vi "Robot Global Data.vi"() -> ()   [LabVIEW 2016]
doc: "This global VI can contain as many global variables as you need. Place a control on the panel, give it a good name. To read or write to it from a VI, drag the icon to the diagram of that VI. You can also drag from the project. Click on the node to change which global you access. You shouldn't have multiple locations writing to a global or it will cause a race-condition."
uses:
  <vilib>/Rock Robotics/WPI/Camera/WPI_CameraImageSize.ctl
  <vilib>/Rock Robotics/WPI/DriverStation/WPI_DriverStationRobotMode2.ctl
panel:
  in  "Robot Enabled":bool
  in  "AutoConstants":T1
  in  "ClimberSpeed":dbl
  in  "IntakeSpeed":dbl
  in  "RightEncoder":dbl
  in  "LeftEncoder":dbl
  in  "Poses":T2(array[cluster])
  in  "Location":cluster{"x":dbl, "y":dbl}
  in  "Angle":dbl
  in  "Diagnostic Message":string
  out "Gear Data":T3
  out "Peg Data":T3
  in  "Vision Target":enum16{"Pegs", "Gears"}(ring)
  in  "RightValue":dbl
  in  "LeftValue":dbl
  in  "ArmState":enum16{"Up", "Down"}(ring)
  in  "PincherState":enum16{"Open", "Close"}(ring)
  in  "Refnums":string[](array[string])
  in  "Robot Mode":T4
  in  "image size":T5=enum."320x240"
  in  "Enable Vision":bool
  # "Drive Base"
  # "Vision"
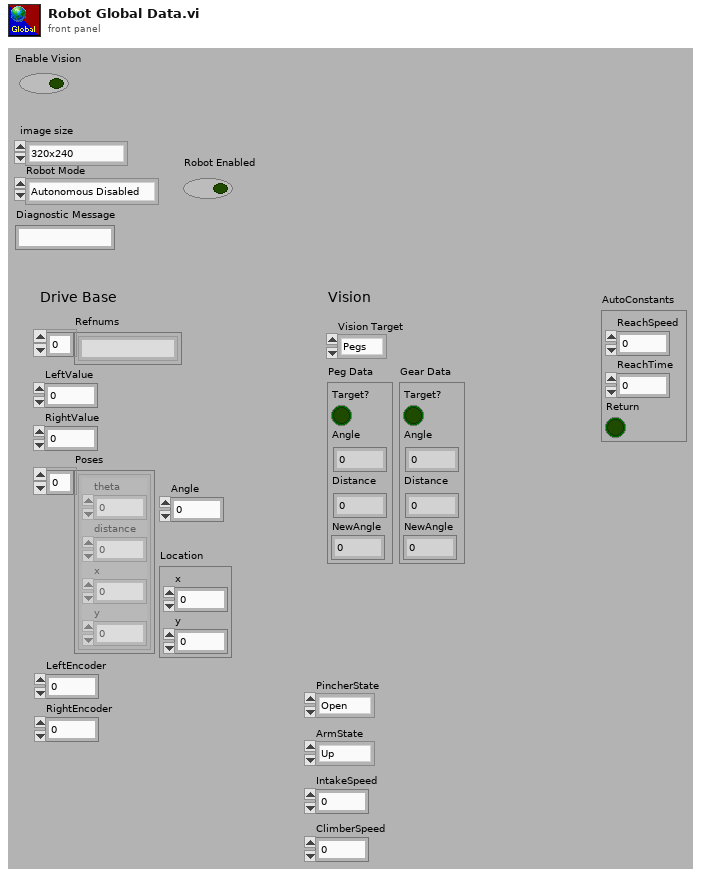
[diagram p1: front panel]
types:
  T1 = cluster{"ReachSpeed":dbl, "ReachTime":dbl, "Return":bool}
  T2 = cluster{"theta":dbl, "distance":dbl, "x":dbl, "y":dbl}[]
  T3 = cluster{"Target?":bool, "Angle":dbl, "Distance":dbl, "NewAngle":dbl}
  T4 = typedef "WPI_DriverStationRobotMode2.ctl" = enum16{"Autonomous Disabled", "Autonomous Enabled", "Teleop Disabled", "Teleop Enabled", "Disconnected", "Finish", "Test Disabled", "Test Enabled", "Emergency Stopped"}
  T5 = typedef "WPI_CameraImageSize.ctl" = enum16{"640x480", "320x240", "160x120", "Custom"}
diagram:
